vi "Write Subset.vi"(8 "error in (no error)":errorcluster, 10 "Subset":cluster{"index":i32, "length":i32}={"index"=0, "length"=100}, 11 "AlicatCommBank in":refnum<class "AlicatCommBank.lvclass">=refnum) -> (0 "error out":errorcluster, 3 "AlicatCommBank out":refnum<class "AlicatCommBank.lvclass">)   [LabVIEW 2014, in "Alicat.lvlib" / "AlicatCommBank.lvclass"]
uses:
  AlicatCommBank.lvclass
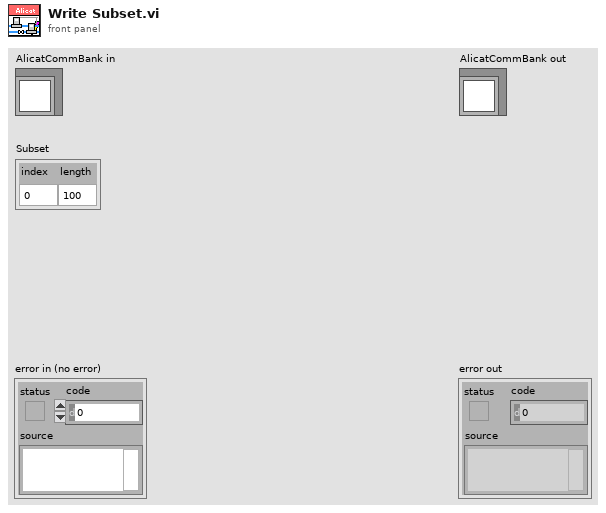
[diagram p1: front panel]
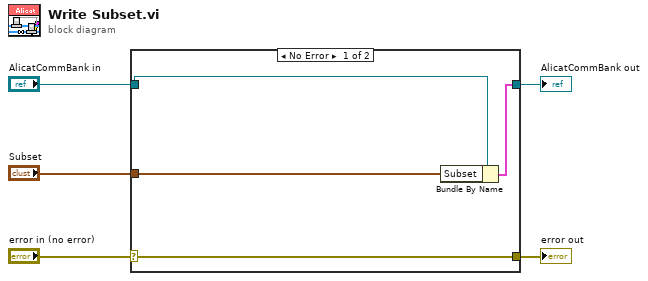
[diagram p0: block diagram]
diagram:
  n1 = case shown="No Error" "error in (no error)" {
    selector: "error in (no error)" -> [w9 w10]
    tunnel: [w9 w10] -> w4
    tunnel: [w7 w11] -> w2
    tunnel: "AlicatCommBank in" -> [w8 w11]
    tunnel: "Subset" -> [w6 _]
    frame No Error {
      n2 = Bundle By Name(cluster=w8, "Subset"=w6) -> (w7:cluster{})
    }
    frame Error {
    }
  }
  "error out" <- w4
  "AlicatCommBank out" <- w2
